vi "Get Class FQN.vi"(10 "LabVIEW Object":refnum<class>) -> (2 "QualifiedName":string)   [LabVIEW 2023, in "Class Loader.lvlib" / "Class Loader.lvclass"]
uses:
  Class Loader.lvclass
  Class Loader.lvclass/Class Loader.ctl
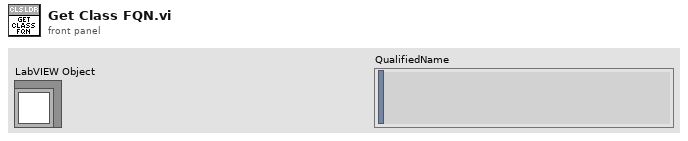
[diagram p1: front panel]
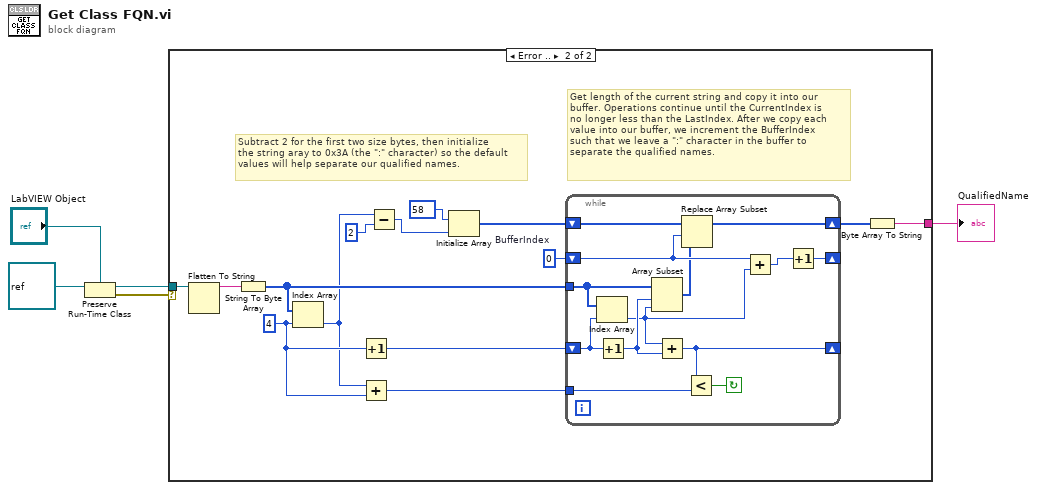
[diagram p0: block diagram]
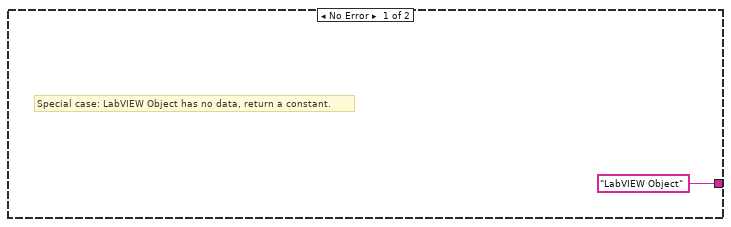
[diagram p2: hidden frame]
diagram:
  n1 = Preserve Run-Time Class(object in=refnum<class> refnum ("LabVIEW Object"), 2:"LabVIEW Object") -> (object out=w2:refnum<class>, error out=w1:errorcluster)  [unwired: 1 in]
  n2 = case shown="Error .." w1 {
    tunnel: w2 -> [_ w9]
    tunnel: ["LabVIEW Object" ("string") w7] -> w5
    frame No Error {
      # "Special case: LabVIEW Object has no data, return a constant."
    }
    frame Error {
      w11 = 0  # BufferIndex
      w18 = 4 ("index")
      # "Get length of the current string and copy it into our\nbuffer. Operations continue until the CurrentIndex is\nno longer less than the LastIndex. After we copy each\nvalue into our buffer, we increment the BufferIndex\nsuch that we leave a \":\" character in the buffer to\nseparate the qualified names."
      # "Subtract 2 for the first two size bytes, then initialize\nthe string aray to 0x3A (the \":\" character) so the default\nvalues will help separate our qualified names."
      n3 = Flatten To String(anything=w9) -> (data string=w10:string)  [unwired: 3 in, 2 out]
      n4 = String To Byte Array(string=w10) -> (unsigned byte array=w20:u8[])
      n5 = Index Array(array=w20, index=w18) -> (element=w16:u8)
      n6 = Increment(x=w18) -> (x+1=w17:i32)
      n7 = Add(x=w16, y=w18) -> (x+y=w19:i32)
      n8 = Subtract(x=w16, y=u8 2) -> (x-y=w14:u8)
      n9 = Initialize Array(u8 58, w14) -> (w12:u8[])
      n10 = while {
        tunnel: w19 -> [w30]
        shift-right: [w31] -> _
        shift-left: w17 -> [w32]
        tunnel: w20 -> [w33]
        shift-right: [w27] -> w8
        shift-left: w12 -> [w28]
        shift-right: [w21] -> _
        shift-left: w11 -> [w25]
        stop <- w29 continue-if-true
        n11 = Index Array(array=w33, index=w32) -> (element=w22:u8)
        n12 = Increment(x=w32) -> (x+1=w26:i32)
        n13 = Array Subset(array=w33, index=w26, length=w22) -> (w23:u8[])
        n14 = Add(x=w22, y=w26) -> (x+y=w31:i32)
        n15 = Replace Array Subset(array=w28, new element=w23, index=w25) -> (w27:u8[])
        n16 = Less?(x=w31, y=w30) -> (x < y?=w29:bool)
        n17 = Add(x=w25, y=w22) -> (x+y=w24:i32)
        n18 = Increment(x=w24) -> (x+1=w21:i32)
      }
      n19 = Byte Array To String(unsigned byte array=w8) -> (string=w7:string)
    }
  }
  "QualifiedName" <- w5
